vi "Teleop.vi"(10 "Match Info":T1={"Autonomous Elapsed Seconds"=0.0, "TeleOp Elapsed Seconds"=0.0, "Disabled Elapsed Seconds"=0.0, "Visited Autonomous"=FALSE, "Visited TeleOp"=FALSE, "Visited Disabled"=FALSE, "Autonomous Settings"={"Autonomous Style"=enum."Independent", "VI Refnum"=refnum}}, 11 "Call Context":T2) -> ()   [LabVIEW 2016]
doc: "This VI is called for each enabled TeleOp packet received from the DS. It is typically used to read from joysticks and other inputs and update I/O or setpoints for timed control loops. It should complete and return within 20 milliseconds or risk missing DS packets."
uses:
  <vilib>/Rock Robotics/WPI/DriverStation/WPI_DriverStationDerivedRobotMode.ctl
  <vilib>/Rock Robotics/WPI/DriverStation/WPI_DriverStationMatch Info.ctl
  AutoTask SubVI/TeleopDrive.ctl
  <vilib>/Rock Robotics/WPI/Solenoid/WPI_SolenoidValue.ctl
  AutoTask/Implementation/AutoTask Setpoints.ctl
  AutoTask/Implementation/AutoTask Operations.ctl
  <vilib>/Rock Robotics/WPI/Utilities/WPI_GetSetVariantRefNum.vi
  <vilib>/Rock Robotics/Network Tables/NT Write Boolean Array.vi
  <vilib>/Rock Robotics/Network Tables/NT Write Numeric Array.vi
  <vilib>/Rock Robotics/Network Tables/NT Read Number.vi
  <vilib>/Rock Robotics/WPI/Solenoid/WPI_SolenoidSetEnum.vi
  NavX/navX Library v2/navX Library v2.lvlib
  <vilib>/Rock Robotics/Network Tables/NT Write Number.vi
panel:
  in  "Driver Control Enable":bool=TRUE
  in  "Drive Beta Enable":bool
  in  "Enable Operator Controls":bool=TRUE
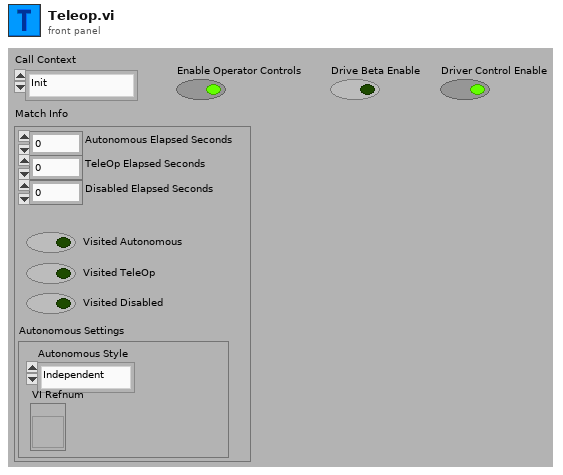
[diagram p1: front panel]
types:
  T1 = typedef "WPI_DriverStationMatch Info.ctl" = cluster{"Autonomous Elapsed Seconds":dbl, "TeleOp Elapsed Seconds":dbl, "Disabled Elapsed Seconds":dbl, "Visited Autonomous":bool, "Visited TeleOp":bool, "Visited Disabled":bool, "Autonomous Settings":cluster{"Autonomous Style":enum16{"Iterative", "Independent"}, "VI Refnum":refnum<vi>}}
  T2 = typedef "WPI_DriverStationDerivedRobotMode.ctl" = enum16{"Init", "Execute", "Stop"}
  T3 = typedef "TeleopDrive.ctl" = enum16{"ToggleLauncher", "StopAgitator", "SetAgitator", "Launch", "Center", "Joystick", "AutoTurn", "AutoAlign", "GearShifter", "Stop", "DriveDistance", "ToggleIntake", "Intake", "AutoIntake"}
  T4 = typedef "WPI_JoystickDevRef.ctl" = cluster{"Device":T5}
  T5 = typedef "WPI_JoystickDeviceEnum.ctl" = enum16{"USB 0", "USB 1", "USB 2", "USB 3", "USB 4", "USB 5"}
  T6 = typedef "WPI_SolenoidValue.ctl" = enum16{"Off", "On", "Forward", "Reverse"}
  T7 = typedef "AutoTask Setpoints.ctl" = cluster{"Operation":T8, "Setpoint":dbl, "Duration":dbl, "Speed":dbl, "Angle":dbl, "VDeadband":dbl, "Deadband":dbl}
  T8 = typedef "AutoTask Operations.ctl" = enum16{"Reserve", "Read Current", "Immediate", "DriveDistance", "AutoShoot", "FaceForward", "AutoAlign", "AutoTurn", "DriveToLine", "DriveToIncline", "DriveTillFlat"}
  T9 = typedef "WPI_SolenoidDevRef.ctl" = cluster{"DevStatus":errorcluster, "Pneumatics Control Module":u8, "Forward Solenoid Channel":T10, "Reverse Solenoid Channel":T10}
  T10 = typedef "WPI_SolenoidChannel.ctl" = enum8{"Solenoid 0", "Solenoid 1", "Solenoid 2", "Solenoid 3", "Solenoid 4", "Solenoid 5", "Solenoid 6", "Solenoid 7", "Invalid"}
  T11 = typedef "navX Library v2.lvlib/Z900_navX_DeviceTypeDef.ctl" = cluster{"Interface":cluster{"Protocol":T12, "Update Rate (4Hz-60Hz)":u8, "navX Open TypeDef":variant}, "Notify Packet":refnum<notifier>, "Loop VI Refnum":refnum<vi>, "Ready to Close Occurrence Refnum":refnum<k4>}
  T12 = typedef "navX Library v2.lvlib/Z900_navX_ProtocolTypeDef.ctl" = enum16{"SERIAL", "I2C", "SPI"}
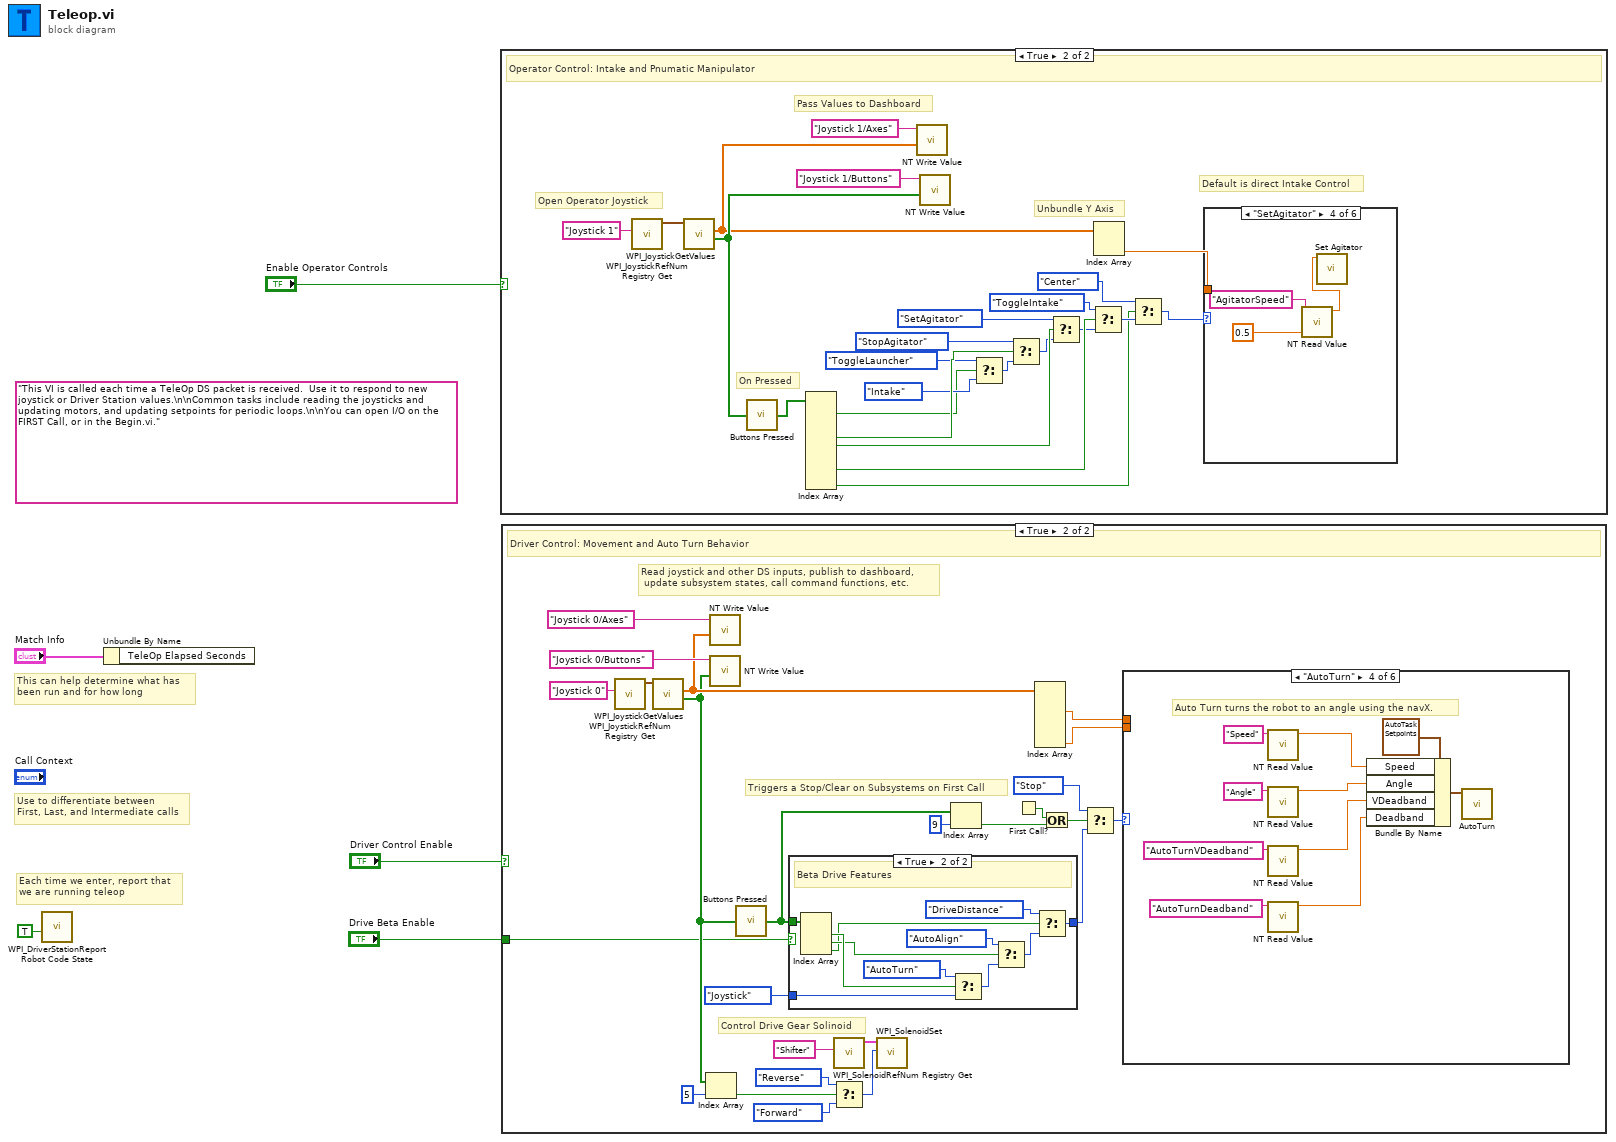
[diagram p0: block diagram]
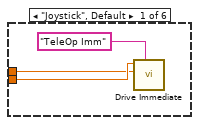
[diagram p4: hidden frame]
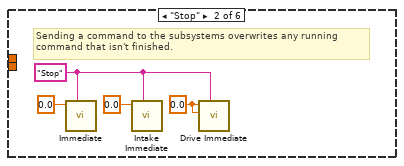
[diagram p5: hidden frame]
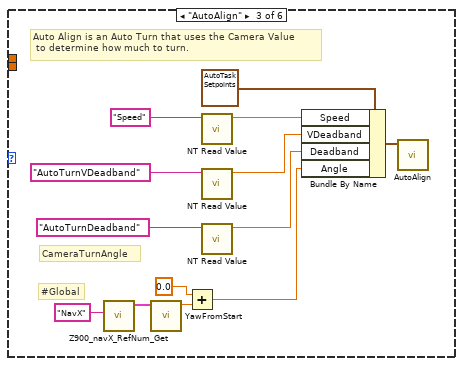
[diagram p6: hidden frame]
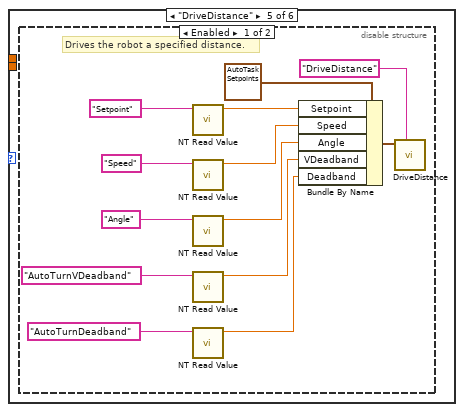
[diagram p7: hidden frame]
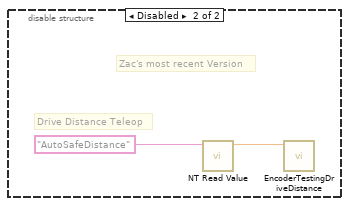
[diagram p8: hidden frame]
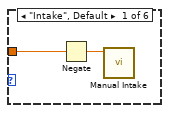
[diagram p11: hidden frame]
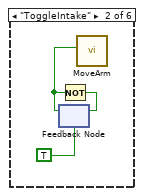
[diagram p12: hidden frame]
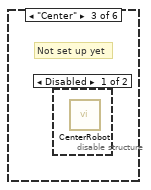
[diagram p13: hidden frame]
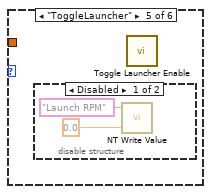
[diagram p15: hidden frame]
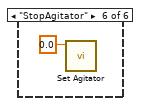
[diagram p17: hidden frame]
diagram:
  (unwired) "This VI is called each time a TeleOp DS packet is received.  Use it to respond to new joystick or Driver Station values.\n\nCommon tasks include reading the joysticks and updating motors, and updating setpoints for periodic loops.\n\nYou can open I/O on the FIRST Call, or in the Begin.vi."
  # "Each time we enter, report that\nwe are running teleop"
  # "Use to differentiate between\nFirst, Last, and Intermediate calls"
  # "This can help determine what has\nbeen run and for how long"
  n1 = call <vilib>:"WPI_DriverStationReport Robot Code State.vi"("TeleOp"=TRUE ("Autonomous")) -> ()  [unwired: 10 in, 1 out]
  n2 = Unbundle By Name("Match Info") -> ()  [unwired: 1 out]
  n3 = case shown="True" "Enable Operator Controls" {
    frame False {
    }
    frame True {
      # "Unbundle Y Axis"
      # "Open Operator Joystick"
      # "Pass Values to Dashboard"
      # "Default is direct Intake Control"
      # "On Pressed"
      # "Operator Control: Intake and Pnumatic Manipulator"
      n4 = call <vilib>:"WPI_JoystickRefNum Registry Get.vi"("refnum name"="Joystick 1") -> ("JoystickDevRef"=w25:T4)  [unwired: 1 in, 9 out]
      n5 = call <vilib>:"WPI_JoystickGetValues.vi"("JoystickDevRef"=w25) -> ("Buttons"=w28:bool[], "Axes"=w23:dbl[])  [unwired: 6 in, 3 out]
      n6 = call "Buttons Pressed.vi"("Button Values"=w28) -> ("Button Presses"=w27:bool[])
      n7 = Index Array(array=w27) -> (element #1=w9:bool, element #4=w13:bool, element #5=w16:bool, element #8=w21:bool, element #10=w18:bool)  [unwired: 10 in, 5 out]
      n8 = call-poly <vilib>:"NT Write Value.vi"("Numeric Array"=w23, "Name"="Joystick 1/Axes") -> ()  [unwired: 9 in, 1 out]
      n9 = call-poly <vilib>:"NT Write Value.vi"("Boolean Array"=w28, "Name"="Joystick 1/Buttons") -> ()  [unwired: 9 in, 1 out]
      n10 = Select(t=TeleopDrive."ToggleLauncher" ("Default Action"), s=w9, f=TeleopDrive."Intake" ("Default Action")) -> (s? t:f=w10:T3)
      n11 = Select(t=TeleopDrive."StopAgitator" ("Default Action"), s=w13, f=w10) -> (s? t:f=w15:T3)
      n12 = Select(t=TeleopDrive."SetAgitator" ("Default Action"), s=w16, f=w15) -> (s? t:f=w7:T3)
      n13 = Select(t=TeleopDrive."ToggleIntake" ("Default Action"), s=w21, f=w7) -> (s? t:f=w20:T3)
      n14 = Index Array(array=w23) -> (element #2=w29:dbl)  [unwired: 2 in, 1 out]
      n15 = Select(t=TeleopDrive."Center" ("Enum"), s=w18, f=w20) -> (s? t:f=w6:T3)
      n16 = case shown="\"SetAgitator\"" w6 {
        tunnel: w29 -> [w31 _ _ _ _ _]
        frame "Intake", Default {
          n17 = Negate(x=w31) -> (-x=w30:dbl)
          n18 = call "Manual Intake.vi"("Setpoint"=w30) -> ()  [unwired: 10 in, 1 out]
        }
        frame "ToggleIntake" {
          n19 = feedback #1(TRUE ("OnOff")) -> (w33:bool)
          n20 = Not(x=w33) -> (.not. x?=w32:bool)
          n21 = feedback-in #1(w32) -> ()
          n22 = call "MoveArm.vi"("OnOff"=w33) -> ()  [unwired: 10 in, 1 out]
        }
        frame "Center" {
          # "Not set up yet"
          n23 = disable-structure shown="Disabled" {
            frame Disabled {
              n24 = call "CenterRobot.vi"() -> ()  [unwired: 11 in, 1 out]
            }
            frame Enabled {
            }
          }
        }
        frame "SetAgitator" {
          n25 = call-poly <vilib>:"NT Read Value.vi"("Default Value"=0.5, "Name"="AgitatorSpeed") -> ("Numeric"=w36:dbl)  [unwired: 8 in, 1 out]
          n26 = call "Set Agitator.vi"("Setpoint"=w36) -> ()  [unwired: 10 in, 1 out]
        }
        frame "ToggleLauncher" {
          n27 = disable-structure shown="Disabled" {
            frame Disabled {
              n28 = call-poly <vilib>:"NT Write Value.vi"("Numeric"=0.0, "Name"="Launch RPM") -> ()  [unwired: 9 in, 1 out]
            }
            frame Enabled {
            }
          }
          n29 = call "Toggle Launcher Enable.vi"() -> ()  [unwired: 11 in, 1 out]
        }
        frame "StopAgitator" {
          n30 = call "Set Agitator.vi"("Setpoint"=0.0) -> ()  [unwired: 10 in, 1 out]
        }
      }
    }
  }
  n31 = case shown="True" "Driver Control Enable" {
    tunnel: "Drive Beta Enable" -> [_ w43]
    frame False {
    }
    frame True {
      # "Triggers a Stop/Clear on Subsystems on First Call"
      # "Control Drive Gear Solinoid"
      # "Read joystick and other DS inputs, publish to dashboard,\n update subsystem states, call command functions, etc."
      # "Driver Control: Movement and Auto Turn Behavior"
      n32 = call <vilib>:"WPI_JoystickRefNum Registry Get.vi"("refnum name"="Joystick 0") -> ("JoystickDevRef"=w64:T4)  [unwired: 1 in, 9 out]
      n33 = call <vilib>:"WPI_JoystickGetValues.vi"("JoystickDevRef"=w64) -> ("Buttons"=w54:bool[], "Axes"=w62:dbl[])  [unwired: 6 in, 3 out]
      n34 = Index Array(array=w54, index=5) -> (element=w48:bool)
      n35 = call-poly <vilib>:"NT Write Value.vi"("Numeric Array"=w62, "Name"="Joystick 0/Axes") -> ()  [unwired: 9 in, 1 out]
      n36 = call-poly <vilib>:"NT Write Value.vi"("Boolean Array"=w54, "Name"="Joystick 0/Buttons") -> ()  [unwired: 9 in, 1 out]
      n37 = call "Buttons Pressed.vi"("Button Values"=w54) -> ("Button Presses"=w45:bool[])
      n38 = case shown="True" w43 {
        tunnel: TeleopDrive."Joystick" ("Enum") -> [w66 w77]
        tunnel: [w66 w73] -> w55
        tunnel: w45 -> [_ w72]
        frame False {
        }
        frame True {
          # "Beta Drive Features"
          n39 = Index Array(array=w72) -> (element #1=w76:bool, element #2=w75:bool, element #3=w74:bool)  [unwired: 3 in]
          n40 = Select(t=TeleopDrive."AutoTurn" ("Enum"), s=w76, f=w77) -> (s? t:f=w70:T3)
          n41 = Select(t=TeleopDrive."AutoAlign" ("Enum"), s=w75, f=w70) -> (s? t:f=w68:T3)
          n42 = Select(t=TeleopDrive."DriveDistance" ("Enum"), s=w74, f=w68) -> (s? t:f=w73:T3)
        }
      }
      n43 = call <vilib>:"WPI_SolenoidRefNum Registry Get.vi"("refnum name"="Shifter") -> ("SolenoidDevRef"=w56:T9)  [unwired: 9 in, 1 out]
      n44 = Select(t=WPI_SolenoidValue."Reverse" ("Value"), s=w48, f=WPI_SolenoidValue."Forward" ("Value")) -> (s? t:f=w47:T6)
      n45 = call-poly <vilib>:"WPI_SolenoidSet.vi"("Value"=w47, "SolenoidDevRef"=w56) -> ()  [unwired: 8 in, 2 out]
      n46 = Index Array(array=w45, index=9) -> (element=w44:bool)
      n47 = First Call?() -> (First Call?: T/F=w52:bool)
      n48 = Index Array(array=w62) -> (element #2=w42:dbl, element #6=w41:dbl)  [unwired: 6 in, 4 out]
      n49 = Or(x=w52, y=w44) -> (x .or. y?=w53:bool)
      n50 = Select(t=TeleopDrive."Stop" ("Enum"), s=w53, f=w55) -> (s? t:f=w58:T3)
      n51 = case shown="\"AutoTurn\"" w58 {
        tunnel: w41 -> [w79 _ _ _ _ _]
        tunnel: w42 -> [w78 _ _ _ _ _]
        frame "Joystick", Default {
          n52 = call "Drive Immediate.vi"("Description"="TeleOp Imm", "Right Setpoint"=w78, "Left Setpoint"=w79) -> ()  [unwired: 8 in, 1 out]
        }
        frame "Stop" {
          w81 = "Stop" ("Description")
          w84 = 0.0
          # "Sending a command to the subsystems overwrites any running\ncommand that isn't finished."
          n53 = call "Immediate.vi"("Description"=w81, "Setpoint"=0.0) -> ()  [unwired: 9 in, 1 out]
          n54 = call "Intake Immediate.vi"("Description"=w81, "Setpoint"=0.0) -> ()  [unwired: 9 in, 1 out]
          n55 = call "Drive Immediate.vi"("Description"=w81, "Right Setpoint"=w84, "Left Setpoint"=w84) -> ()  [unwired: 8 in, 1 out]
        }
        frame "AutoAlign" {
          # "#Global"
          # "CameraTurnAngle"
          # "Auto Align is an Auto Turn that uses the Camera Value\n to determine how much to turn."
          n56 = call "Z900_navX_RefNum_Get.vi"("refnum name"="NavX") -> ("navX Device"=w95:T11)  [unwired: 9 in, 1 out]
          n57 = call "YawFromStart.vi"("navX Device"=w95) -> ("Yaw"=w96:dbl)  [unwired: 10 in]
          n58 = Add(x=0.0, y=w96) -> (x+y=w97:dbl)
          n59 = call-poly <vilib>:"NT Read Value.vi"("Name"="Speed") -> ("Numeric"=w93:dbl)  [unwired: 9 in, 1 out]
          n60 = call-poly <vilib>:"NT Read Value.vi"("Name"="AutoTurnVDeadband") -> ("Numeric"=w89:dbl)  [unwired: 9 in, 1 out]
          n61 = call-poly <vilib>:"NT Read Value.vi"("Name"="AutoTurnDeadband") -> ("Numeric"=w91:dbl)  [unwired: 9 in, 1 out]
          n62 = Bundle By Name(cluster=T7 {"Operation"=enum."AutoAlign", "Setpoint"=0.0, "Duration"=0.0, "Speed"=0.0, "Angle"=0.0, "VDeadband"=0.0, "Deadband"=0.0} ("SubSystem Data"), "Speed"=w93, "VDeadband"=w89, "Deadband"=w91, "Angle"=w97) -> (w86:T7)
          n63 = call "AutoAlign.vi"("SubSystem Data"=w86) -> ()  [unwired: 10 in, 1 out]
        }
        frame "AutoTurn" {
          # "Auto Turn turns the robot to an angle using the navX."
          n64 = call-poly <vilib>:"NT Read Value.vi"("Name"="Speed") -> ("Numeric"=w100:dbl)  [unwired: 9 in, 1 out]
          n65 = call-poly <vilib>:"NT Read Value.vi"("Name"="Angle") -> ("Numeric"=w102:dbl)  [unwired: 9 in, 1 out]
          n66 = call-poly <vilib>:"NT Read Value.vi"("Name"="AutoTurnVDeadband") -> ("Numeric"=w106:dbl)  [unwired: 9 in, 1 out]
          n67 = call-poly <vilib>:"NT Read Value.vi"("Name"="AutoTurnDeadband") -> ("Numeric"=w104:dbl)  [unwired: 9 in, 1 out]
          n68 = Bundle By Name(cluster=T7 {"Operation"=enum."AutoTurn", "Setpoint"=0.0, "Duration"=0.0, "Speed"=0.0, "Angle"=0.0, "VDeadband"=0.0, "Deadband"=0.0} ("SubSystem Data"), "Speed"=w100, "Angle"=w102, "VDeadband"=w106, "Deadband"=w104) -> (w107:T7)
          n69 = call "AutoTurn.vi"("SubSystem Data"=w107) -> ()  [unwired: 9 in, 1 out]
        }
        frame "DriveDistance" {
          n70 = disable-structure shown="Enabled" {
            frame Enabled {
              # "Drives the robot a specified distance."
              n71 = call-poly <vilib>:"NT Read Value.vi"("Name"="Setpoint") -> ("Numeric"=w117:dbl)  [unwired: 9 in, 1 out]
              n72 = call-poly <vilib>:"NT Read Value.vi"("Name"="Speed") -> ("Numeric"=w111:dbl)  [unwired: 9 in, 1 out]
              n73 = call-poly <vilib>:"NT Read Value.vi"("Name"="Angle") -> ("Numeric"=w113:dbl)  [unwired: 9 in, 1 out]
              n74 = call-poly <vilib>:"NT Read Value.vi"("Name"="AutoTurnVDeadband") -> ("Numeric"=w119:dbl)  [unwired: 9 in, 1 out]
              n75 = call-poly <vilib>:"NT Read Value.vi"("Name"="AutoTurnDeadband") -> ("Numeric"=w115:dbl)  [unwired: 9 in, 1 out]
              n76 = Bundle By Name(cluster=T7 {"Operation"=enum."DriveDistance", "Setpoint"=0.0, "Duration"=0.0, "Speed"=0.0, "Angle"=0.0, "VDeadband"=0.0, "Deadband"=0.0} ("SubSystem Data"), "Setpoint"=w117, "Speed"=w111, "Angle"=w113, "VDeadband"=w119, "Deadband"=w115) -> (w120:T7)
              n77 = call "DriveDistance.vi"("Description"="DriveDistance", "SubSystem Data"=w120) -> ()  [unwired: 9 in, 1 out]
            }
            frame Disabled {
              # "Zac's most recent Version"
              # "Drive Distance Teleop"
              n78 = call-poly <vilib>:"NT Read Value.vi"("Name"="AutoSafeDistance") -> ("Numeric"=w121:dbl)  [unwired: 9 in, 1 out]
              n79 = call "EncoderTestingDriveDistance.vi"("Distance"=w121) -> ()  [unwired: 11 in]
            }
          }
        }
        frame "GearShifter" {
        }
      }
    }
  }
